vi "GDFreadData.vi"(0 "GDFv1.x.lvclass in":refnum<class "GDFv1.x.lvclass">, 9 "Channel Number":i64, 11 "error in":errorcluster) -> (4 "GDFv1.x.lvclass out":refnum<class "GDFv1.x.lvclass">, 6 "waveform out":waveform(dbl), 15 "error out":errorcluster)   [LabVIEW 2016, in "GDF File Reader.lvlib" / "GDFv1.x.lvclass"]
uses:
  GDFv1.x.lvclass
  GDFv1.x.lvclass/GDFv1.x.ctl
panel:
  # "This VI is a part of BCI Design library, http://www.ru-bci.org \nCopyright © 2020, Sotnikov Peter, All rights reserved. License: CC BY-NC 4.0"
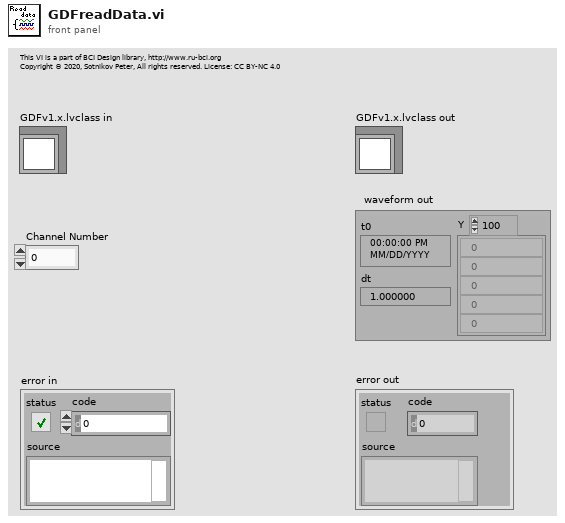
[diagram p1: front panel]
types:
  T1 = typedef "GDF File Reader.lvlib/GdfHeader1.ctl" = cluster{"Version identificator":string, "Patient identificator":string, "Recording identificator":string, "StartDateTime":timestamp, "Header record length":i64, "Equipment Provider":u64, "Laboratory":u64, "Technician":u64, "Number of data records":i64, "Duration of a data record":cluster{"Numerator":u32, "Denominator":u32}, "Number of signals":u32}
  T2 = typedef "GDF File Reader.lvlib/GdfHeader2.ctl" = cluster{"Channel labels":string[], "Transduser types":string[], "Physical dimensions":string[], "Physical lows":dbl[], "Physical highs":dbl[], "Digital lows":dbl[], "Digital highs":dbl[], "Channels Pre-filtering":string[], "Number of samples":u32[], "Channel types":u32[], "Addons":string[]}
  T3 = enum16{"big-endian, network order", "native, host order", "little-endian"}
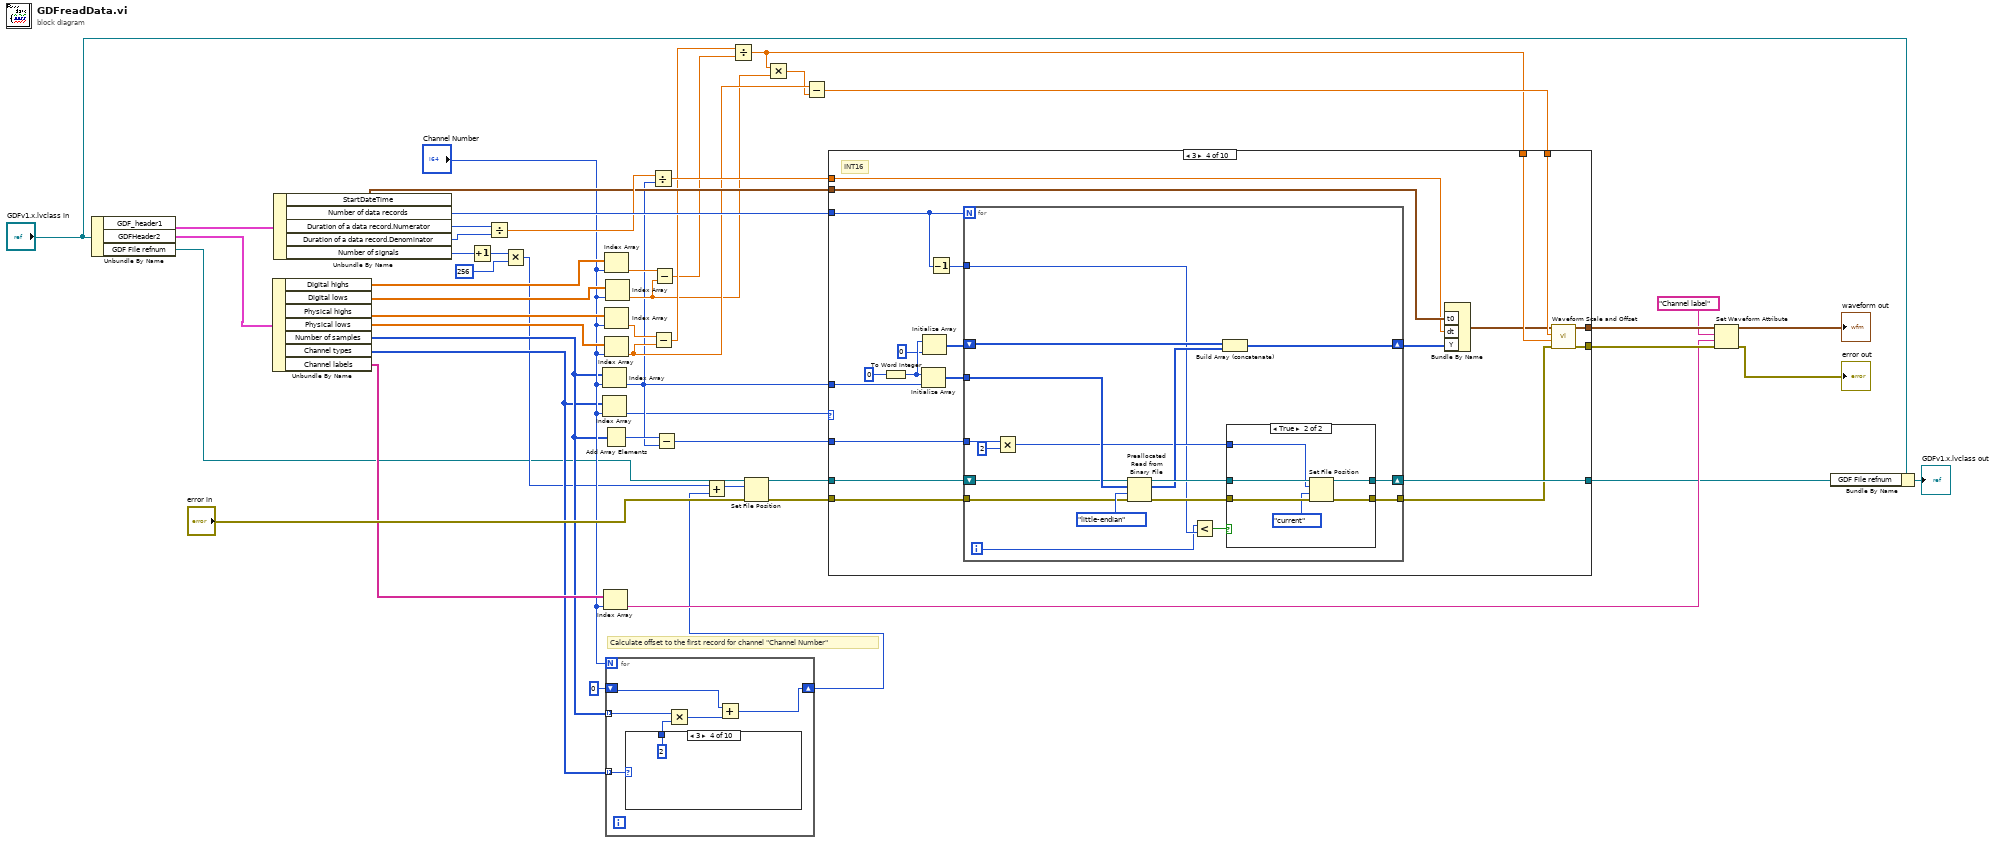
[diagram p0: block diagram]
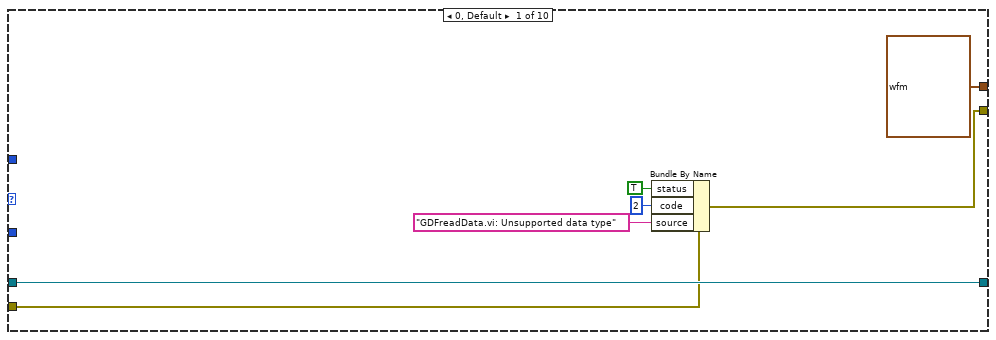
[diagram p2: hidden frame]
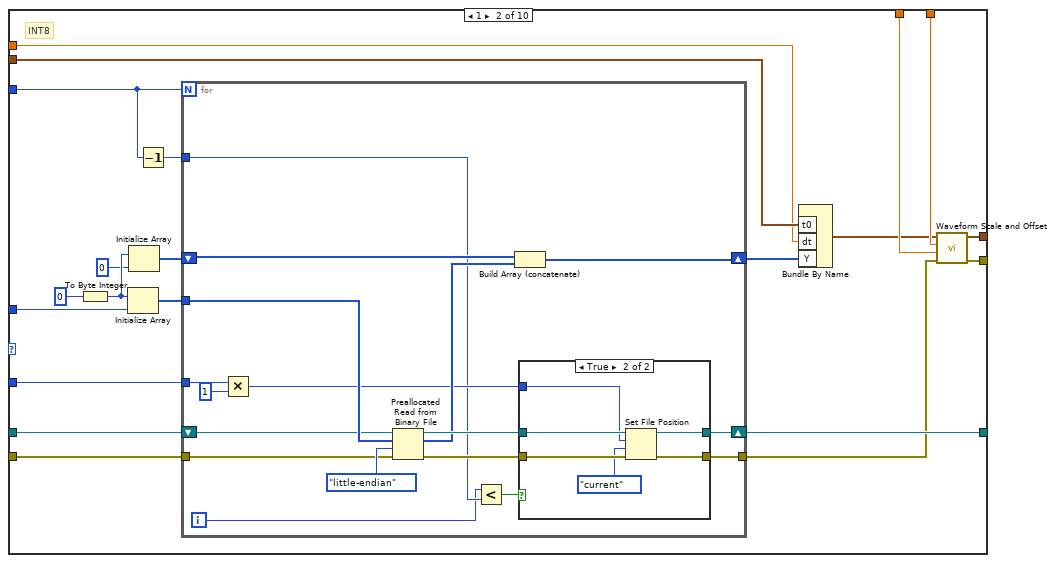
[diagram p3: hidden frame]
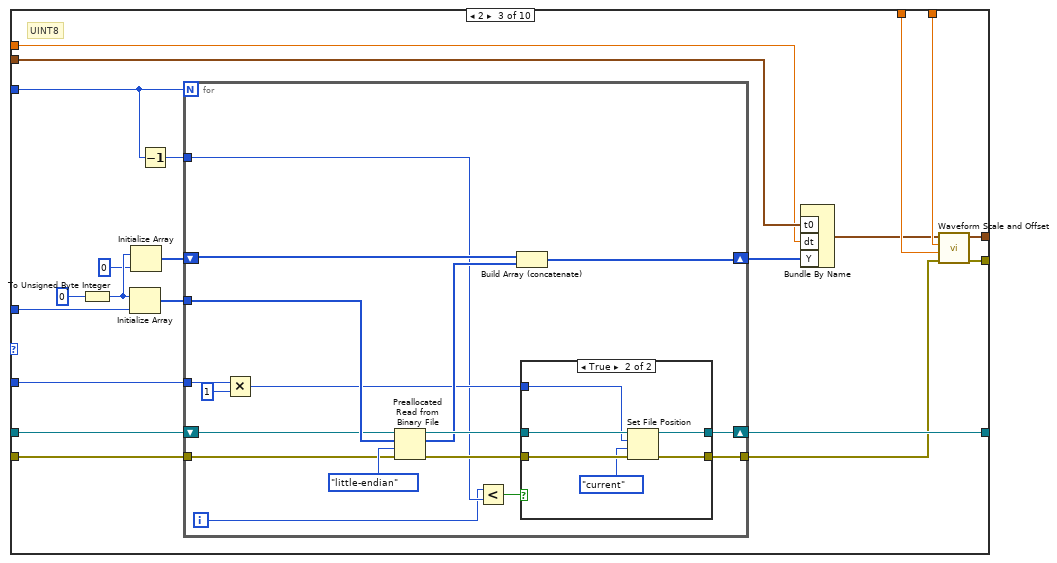
[diagram p5: hidden frame]
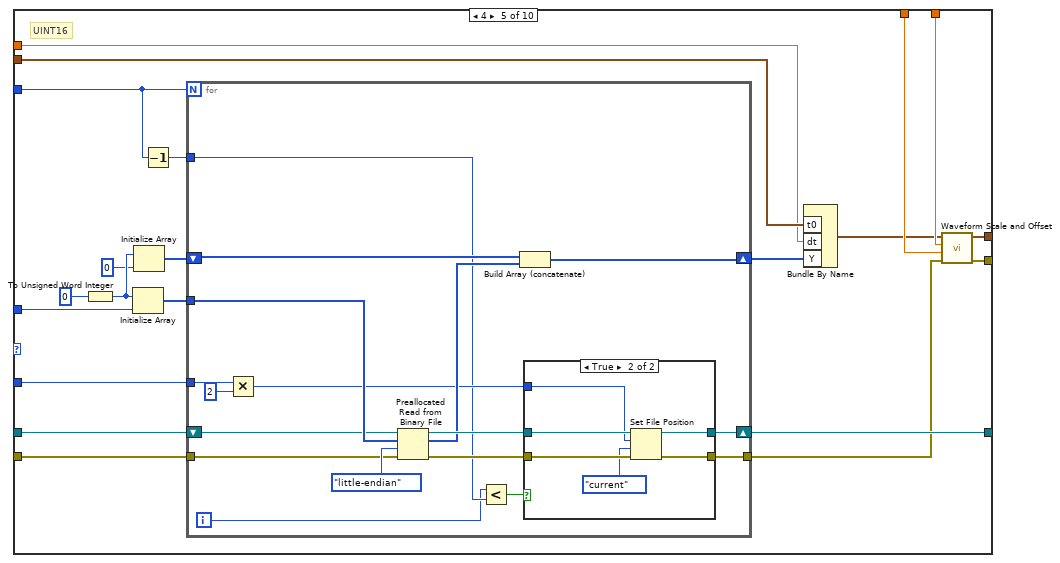
[diagram p8: hidden frame]
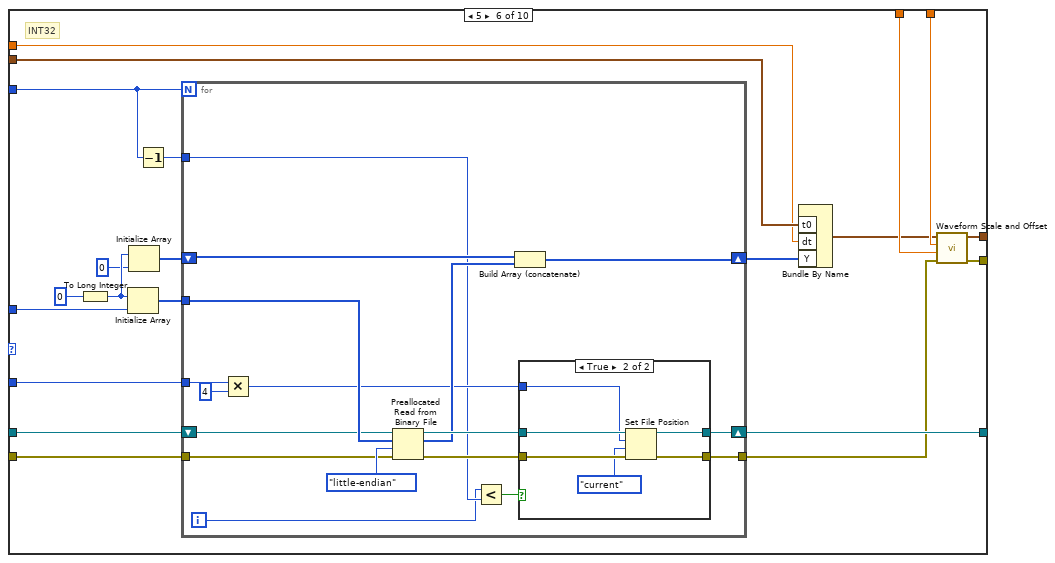
[diagram p10: hidden frame]
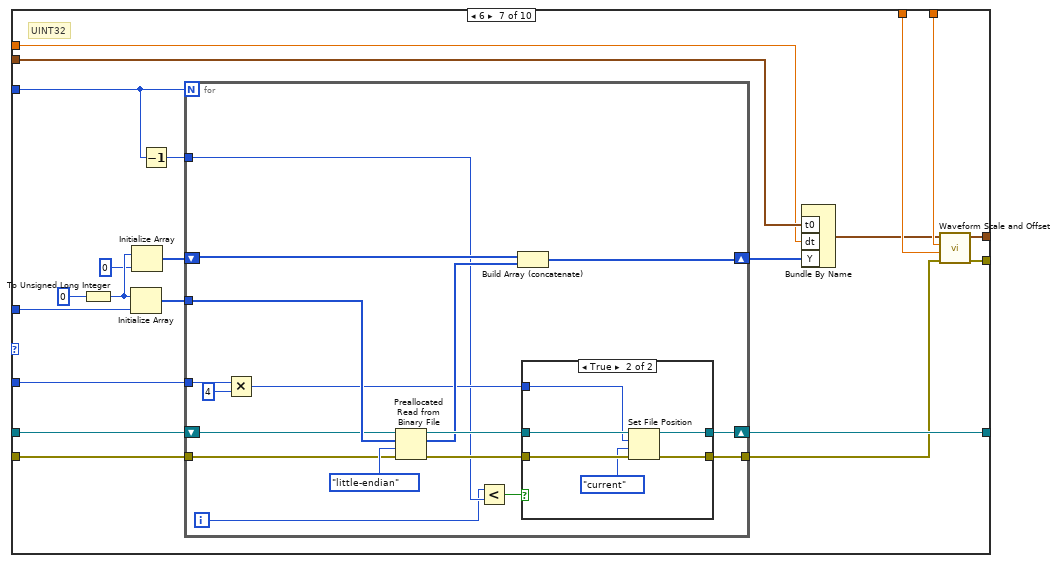
[diagram p12: hidden frame]
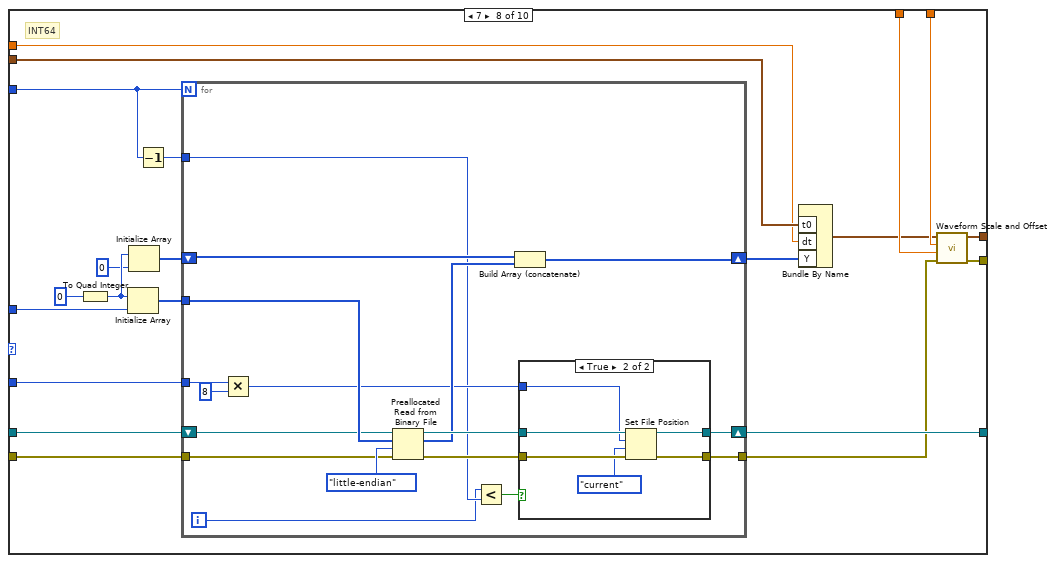
[diagram p14: hidden frame]
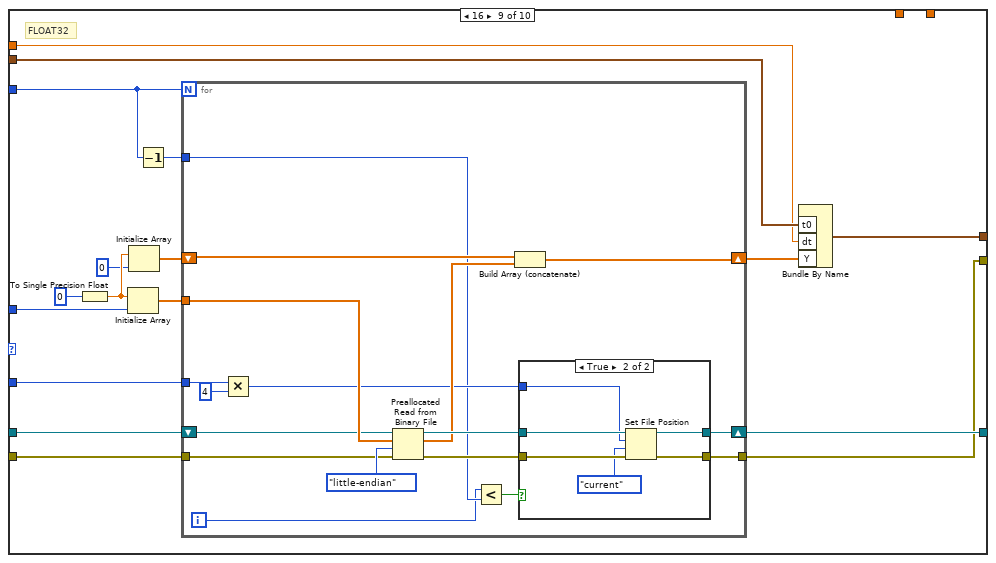
[diagram p16: hidden frame]
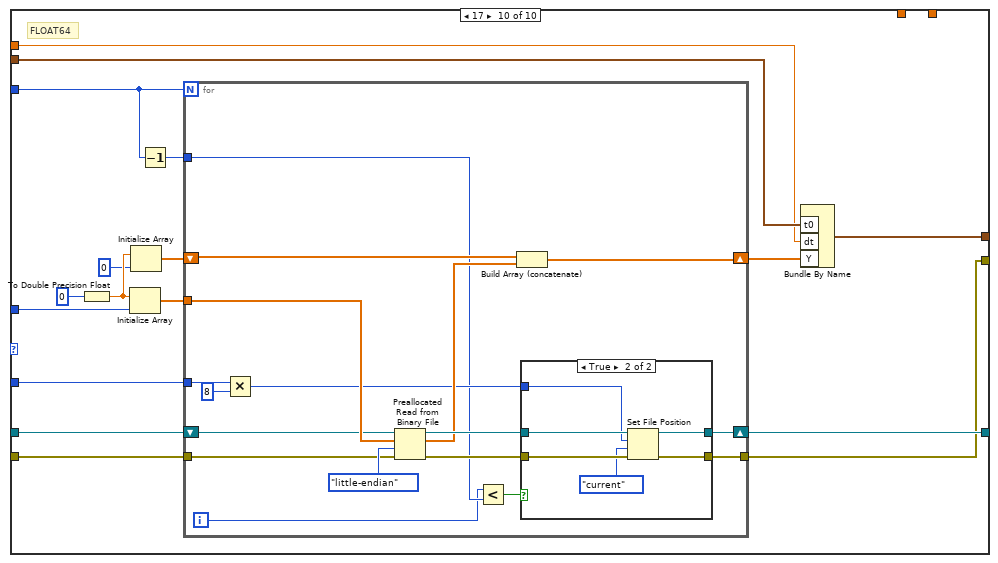
[diagram p18: hidden frame]
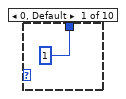
[diagram p20: hidden frame]
diagram:
  # "Calculate offset to the first record for channel \"Channel Number\""
  n1 = Unbundle By Name("GDFv1.x.lvclass in") -> ("GDF_header1"=w6:T1, "GDFHeader2"=w5:T2, "GDF File refnum"=w4:refnum<file>)
  n2 = Unbundle By Name(w5) -> ("Digital highs"=w43:dbl[], "Digital lows"=w33:dbl[], "Physical highs"=w44:dbl[], "Physical lows"=w45:dbl[], "Number of samples"=w14:u32[], "Channel types"=w13:u32[], "Channel labels"=w18:string[])
  n3 = Unbundle By Name(w6) -> ("StartDateTime"=w36:timestamp, "Number of data records"=w46:i64, "Duration of a data record.Numerator"=w39:u32, "Duration of a data record.Denominator"=w38:u32, "Number of signals"=w47:u32)
  n4 = Increment(x=w47) -> (x+1=w49:u32)
  n5 = Divide(x=w39, y=w38) -> (x/y=w37:dbl)
  n6 = Multiply(x=w49, y=u32 256) -> (x*y=w11:u32)
  n7 = Index Array(array=w14, index="Channel Number") -> (element=w23:u32)
  n8 = Index Array(array=w13, index="Channel Number") -> (element=w7:u32)
  n9 = Index Array(array=w18, index="Channel Number") -> (element=w17:string)
  n10 = Index Array(array=w45, index="Channel Number") -> (element=w29:dbl)
  n11 = Add Array Elements(numeric array=w14) -> (sum=w24:u32)
  n12 = Index Array(array=w43, index="Channel Number") -> (element=w32:dbl)
  n13 = Index Array(array=w44, index="Channel Number") -> (element=w34:dbl)
  n14 = Index Array(array=w33, index="Channel Number") -> (element=w27:dbl)
  n15 = for {
    N: "Channel Number" -> [_]
    tunnel: w14 -> [w54] mode=indexing
    tunnel: w13 -> [w55] mode=indexing
    shift-right: [w50] -> w10
    shift-left: u32 0 -> [w51]
    n16 = case shown="3" w55 {
      tunnel: [1 1 1 2 2 4 4 8 4 8] -> w53
      frame 0, Default {
      }
      frame 1 {
      }
      frame 2 {
      }
      frame 3 {
      }
      frame 4 {
      }
      frame 5 {
      }
      frame 6 {
      }
      frame 7 {
      }
      frame 16 {
      }
      frame 17 {
      }
    }
    n17 = Multiply(x=w54, y=w53) -> (x*y=w52:u32)
    n18 = Add(x=w51, y=w52) -> (x+y=w50:u32)
  }
  n19 = Divide(x=w37, y=w23) -> (x/y=w35:dbl)
  n20 = Subtract(x=w34, y=w29) -> (x-y=w31:dbl)
  n21 = Subtract(x=w32, y=w27) -> (x-y=w30:dbl)
  n22 = Subtract(x=w24, y=w23) -> (x-y=w22:u32)
  n23 = Add(x=w11, y=w10) -> (x+y=w9:u32)
  n24 = Divide(x=w31, y=w30) -> (x/y=w25:dbl)
  n25 = Set File Position(offset (in bytes) (0)=w9, refnum=w4, error in="error in") -> (refnum out=w40:refnum<file>, error out=w41:errorcluster)  [unwired: 1 in]
  n26 = Multiply(x=w25, y=w27) -> (x*y=w28:dbl)
  n27 = Subtract(x=w29, y=w28) -> (x-y=w26:dbl)
  n28 = case shown="3" w7 {
    tunnel: w46 -> [_ w93 w139 w185 w231 w277 w323 w369 w411 w453]
    tunnel: w41 -> [w70 w92 w138 w184 w230 w276 w322 w368 w410 w452]
    tunnel: w40 -> [w71 w91 w137 w183 w229 w275 w321 w367 w409 w451]
    tunnel: [w71 w90 w136 w182 w228 w274 w320 w366 w408 w450] -> w2
    tunnel: w36 -> [_ w89 w135 w181 w227 w273 w319 w365 w407 w449]
    tunnel: w35 -> [_ w88 w134 w180 w226 w272 w318 w364 w406 w448]
    tunnel: w26 -> [_ w87 w133 w179 w225 w271 w317 w363 _ _]
    tunnel: w25 -> [_ w86 w132 w178 w224 w270 w316 w362 _ _]
    tunnel: w23 -> [_ w85 w131 w177 w223 w269 w315 w361 w405 w447]
    tunnel: w22 -> [_ w84 w130 w176 w222 w268 w314 w360 w404 w446]
    tunnel: [waveform(dbl) {"t0"=timestamp(0 s since 1904-01-01), "dt"=1.0, "Y"=[]} ("waveform out") w83 w129 w175 w221 w267 w313 w359 w396 w438] -> w21
    tunnel: [w69 w82 w128 w174 w220 w266 w312 w358 w395 w437] -> w20
    frame 0, Default {
      n29 = Bundle By Name(cluster=w70, "status"=TRUE, "code"=2, "source"="GDFreadData.vi: Unsupported data type") -> (w69:errorcluster)
    }
    frame 1 {
      # "INT8"
      n30 = To Byte Integer(number=i16 0) -> (8bit integer=w77:i8)
      n31 = Initialize Array(w77, w85) -> (w78:i8[])
      n32 = Initialize Array(w77, 0 ("dimension size")) -> (w76:i8[])
      n33 = Decrement(x=w93) -> (x-1=w73:i64)
      n34 = for {
        N: w93 -> [_]
        tunnel: w78 -> [w110]
        tunnel: w92 -> [w108]
        tunnel: [w104] -> w80
        shift-right: [w103] -> w90
        shift-left: w91 -> [w107]
        shift-right: [w101] -> w74
        shift-left: w76 -> [w100]
        tunnel: w84 -> [w99]
        tunnel: w73 -> [w95]
        i -> [w94]
        n35 = Multiply(x=w99, y=u32 1) -> (x*y=w97:u32)
        n36 = Preallocated Read from Binary File(4:w108, 5:T3."little-endian" ("byte order (0:big-endian, network order)"), 6:w110, 7:w107) -> (0:w106:errorcluster, 2:w102:i8[], 3:w105:refnum<file>)  [unwired: 1 out]
        n37 = Less?(x=w94, y=w95) -> (x < y?=w96:bool)
        n38 = Build Array (concatenate)(w100, w102) -> (w101:i8[])
        n39 = case shown="True" w96 {
          tunnel: w106 -> [w111 w118]
          tunnel: w105 -> [w112 w117]
          tunnel: [w111 w115] -> w104
          tunnel: [w112 w114] -> w103
          tunnel: w97 -> [_ w113]
          frame False {
          }
          frame True {
            n40 = Set File Position(offset (in bytes) (0)=w113, refnum=w117, from (0:start)=enum16{"start", "end", "current"}."current", error in=w118) -> (refnum out=w114:refnum<file>, error out=w115:errorcluster)
          }
        }
      }
      n41 = Bundle By Name("t0"=w89, "dt"=w88, "Y"=w74) -> (w81:waveform(i8))  [unwired: 1 in]
      n42 = call <vilib>:"Waveform Scale and Offset.vi"("error in (no error)"=w80, "scale"=w86, "offset"=w87, "waveform in"=w81) -> ("error out"=w82:errorcluster, "waveform out"=w83:waveform(dbl))  [unwired: 6 in]
    }
    frame 2 {
      # "UINT8"
      n43 = To Unsigned Byte Integer(number=i16 0) -> (unsigned 8bit integer=w123:u8)
      n44 = Initialize Array(w123, w131) -> (w124:u8[])
      n45 = Initialize Array(w123, 0 ("dimension size")) -> (w122:u8[])
      n46 = Decrement(x=w139) -> (x-1=w119:i64)
      n47 = for {
        N: w139 -> [_]
        tunnel: w124 -> [w156]
        tunnel: w138 -> [w154]
        tunnel: [w150] -> w126
        shift-right: [w149] -> w136
        shift-left: w137 -> [w153]
        shift-right: [w147] -> w120
        shift-left: w122 -> [w146]
        tunnel: w130 -> [w145]
        tunnel: w119 -> [w141]
        i -> [w140]
        n48 = Multiply(x=w145, y=u32 1) -> (x*y=w143:u32)
        n49 = Preallocated Read from Binary File(4:w154, 5:T3."little-endian" ("byte order (0:big-endian, network order)"), 6:w156, 7:w153) -> (0:w152:errorcluster, 2:w148:u8[], 3:w151:refnum<file>)  [unwired: 1 out]
        n50 = Less?(x=w140, y=w141) -> (x < y?=w142:bool)
        n51 = Build Array (concatenate)(w146, w148) -> (w147:u8[])
        n52 = case shown="True" w142 {
          tunnel: w152 -> [w157 w164]
          tunnel: w151 -> [w158 w163]
          tunnel: [w157 w161] -> w150
          tunnel: [w158 w160] -> w149
          tunnel: w143 -> [_ w159]
          frame False {
          }
          frame True {
            n53 = Set File Position(offset (in bytes) (0)=w159, refnum=w163, from (0:start)=enum16{"start", "end", "current"}."current", error in=w164) -> (refnum out=w160:refnum<file>, error out=w161:errorcluster)
          }
        }
      }
      n54 = Bundle By Name("t0"=w135, "dt"=w134, "Y"=w120) -> (w127:waveform(u8))  [unwired: 1 in]
      n55 = call <vilib>:"Waveform Scale and Offset.vi"("error in (no error)"=w126, "scale"=w132, "offset"=w133, "waveform in"=w127) -> ("error out"=w128:errorcluster, "waveform out"=w129:waveform(dbl))  [unwired: 6 in]
    }
    frame 3 {
      # "INT16"
      n56 = To Word Integer(number=i16 0) -> (16bit integer=w169:i16)
      n57 = Initialize Array(w169, w177) -> (w170:i16[])
      n58 = Initialize Array(w169, 0 ("dimension size")) -> (w168:i16[])
      n59 = Decrement(x=w185) -> (x-1=w165:i64)
      n60 = for {
        N: w185 -> [_]
        tunnel: w170 -> [w202]
        tunnel: w184 -> [w200]
        tunnel: [w196] -> w172
        shift-right: [w195] -> w182
        shift-left: w183 -> [w199]
        shift-right: [w193] -> w166
        shift-left: w168 -> [w192]
        tunnel: w176 -> [w191]
        tunnel: w165 -> [w187]
        i -> [w186]
        n61 = Multiply(x=w191, y=u32 2) -> (x*y=w189:u32)
        n62 = Preallocated Read from Binary File(4:w200, 5:T3."little-endian" ("byte order (0:big-endian, network order)"), 6:w202, 7:w199) -> (0:w198:errorcluster, 2:w194:i16[], 3:w197:refnum<file>)  [unwired: 1 out]
        n63 = Less?(x=w186, y=w187) -> (x < y?=w188:bool)
        n64 = Build Array (concatenate)(w192, w194) -> (w193:i16[])
        n65 = case shown="True" w188 {
          tunnel: w198 -> [w203 w210]
          tunnel: w197 -> [w204 w209]
          tunnel: [w203 w207] -> w196
          tunnel: [w204 w206] -> w195
          tunnel: w189 -> [_ w205]
          frame False {
          }
          frame True {
            n66 = Set File Position(offset (in bytes) (0)=w205, refnum=w209, from (0:start)=enum16{"start", "end", "current"}."current", error in=w210) -> (refnum out=w206:refnum<file>, error out=w207:errorcluster)
          }
        }
      }
      n67 = Bundle By Name("t0"=w181, "dt"=w180, "Y"=w166) -> (w173:waveform(i16))  [unwired: 1 in]
      n68 = call <vilib>:"Waveform Scale and Offset.vi"("error in (no error)"=w172, "scale"=w178, "offset"=w179, "waveform in"=w173) -> ("error out"=w174:errorcluster, "waveform out"=w175:waveform(dbl))  [unwired: 6 in]
    }
    frame 4 {
      # "UINT16"
      n69 = To Unsigned Word Integer(number=i16 0) -> (unsigned 16bit integer=w215:u16)
      n70 = Initialize Array(w215, w223) -> (w216:u16[])
      n71 = Initialize Array(w215, 0 ("dimension size")) -> (w214:u16[])
      n72 = Decrement(x=w231) -> (x-1=w211:i64)
      n73 = for {
        N: w231 -> [_]
        tunnel: w216 -> [w248]
        tunnel: w230 -> [w246]
        tunnel: [w242] -> w218
        shift-right: [w241] -> w228
        shift-left: w229 -> [w245]
        shift-right: [w239] -> w212
        shift-left: w214 -> [w238]
        tunnel: w222 -> [w237]
        tunnel: w211 -> [w233]
        i -> [w232]
        n74 = Multiply(x=w237, y=u32 2) -> (x*y=w235:u32)
        n75 = Preallocated Read from Binary File(4:w246, 5:T3."little-endian" ("byte order (0:big-endian, network order)"), 6:w248, 7:w245) -> (0:w244:errorcluster, 2:w240:u16[], 3:w243:refnum<file>)  [unwired: 1 out]
        n76 = Less?(x=w232, y=w233) -> (x < y?=w234:bool)
        n77 = Build Array (concatenate)(w238, w240) -> (w239:u16[])
        n78 = case shown="True" w234 {
          tunnel: w244 -> [w249 w256]
          tunnel: w243 -> [w250 w255]
          tunnel: [w249 w253] -> w242
          tunnel: [w250 w252] -> w241
          tunnel: w235 -> [_ w251]
          frame False {
          }
          frame True {
            n79 = Set File Position(offset (in bytes) (0)=w251, refnum=w255, from (0:start)=enum16{"start", "end", "current"}."current", error in=w256) -> (refnum out=w252:refnum<file>, error out=w253:errorcluster)
          }
        }
      }
      n80 = Bundle By Name("t0"=w227, "dt"=w226, "Y"=w212) -> (w219:waveform(u16))  [unwired: 1 in]
      n81 = call <vilib>:"Waveform Scale and Offset.vi"("error in (no error)"=w218, "scale"=w224, "offset"=w225, "waveform in"=w219) -> ("error out"=w220:errorcluster, "waveform out"=w221:waveform(dbl))  [unwired: 6 in]
    }
    frame 5 {
      # "INT32"
      n82 = To Long Integer(number=i16 0) -> (32bit integer=w261:i32)
      n83 = Initialize Array(w261, w269) -> (w262:i32[])
      n84 = Initialize Array(w261, 0 ("dimension size")) -> (w260:i32[])
      n85 = Decrement(x=w277) -> (x-1=w257:i64)
      n86 = for {
        N: w277 -> [_]
        tunnel: w262 -> [w294]
        tunnel: w276 -> [w292]
        tunnel: [w288] -> w264
        shift-right: [w287] -> w274
        shift-left: w275 -> [w291]
        shift-right: [w285] -> w258
        shift-left: w260 -> [w284]
        tunnel: w268 -> [w283]
        tunnel: w257 -> [w279]
        i -> [w278]
        n87 = Multiply(x=w283, y=u32 4) -> (x*y=w281:u32)
        n88 = Preallocated Read from Binary File(4:w292, 5:T3."little-endian" ("byte order (0:big-endian, network order)"), 6:w294, 7:w291) -> (0:w290:errorcluster, 2:w286:i32[], 3:w289:refnum<file>)  [unwired: 1 out]
        n89 = Less?(x=w278, y=w279) -> (x < y?=w280:bool)
        n90 = Build Array (concatenate)(w284, w286) -> (w285:i32[])
        n91 = case shown="True" w280 {
          tunnel: w290 -> [w295 w302]
          tunnel: w289 -> [w296 w301]
          tunnel: [w295 w299] -> w288
          tunnel: [w296 w298] -> w287
          tunnel: w281 -> [_ w297]
          frame False {
          }
          frame True {
            n92 = Set File Position(offset (in bytes) (0)=w297, refnum=w301, from (0:start)=enum16{"start", "end", "current"}."current", error in=w302) -> (refnum out=w298:refnum<file>, error out=w299:errorcluster)
          }
        }
      }
      n93 = Bundle By Name("t0"=w273, "dt"=w272, "Y"=w258) -> (w265:waveform(i32))  [unwired: 1 in]
      n94 = call <vilib>:"Waveform Scale and Offset.vi"("error in (no error)"=w264, "scale"=w270, "offset"=w271, "waveform in"=w265) -> ("error out"=w266:errorcluster, "waveform out"=w267:waveform(dbl))  [unwired: 6 in]
    }
    frame 6 {
      # "UINT32"
      n95 = To Unsigned Long Integer(number=i16 0) -> (unsigned 32bit integer=w307:u32)
      n96 = Initialize Array(w307, w315) -> (w308:u32[])
      n97 = Initialize Array(w307, 0 ("dimension size")) -> (w306:u32[])
      n98 = Decrement(x=w323) -> (x-1=w303:i64)
      n99 = for {
        N: w323 -> [_]
        tunnel: w308 -> [w340]
        tunnel: w322 -> [w338]
        tunnel: [w334] -> w310
        shift-right: [w333] -> w320
        shift-left: w321 -> [w337]
        shift-right: [w331] -> w304
        shift-left: w306 -> [w330]
        tunnel: w314 -> [w329]
        tunnel: w303 -> [w325]
        i -> [w324]
        n100 = Multiply(x=w329, y=u32 4) -> (x*y=w327:u32)
        n101 = Preallocated Read from Binary File(4:w338, 5:T3."little-endian" ("byte order (0:big-endian, network order)"), 6:w340, 7:w337) -> (0:w336:errorcluster, 2:w332:u32[], 3:w335:refnum<file>)  [unwired: 1 out]
        n102 = Less?(x=w324, y=w325) -> (x < y?=w326:bool)
        n103 = Build Array (concatenate)(w330, w332) -> (w331:u32[])
        n104 = case shown="True" w326 {
          tunnel: w336 -> [w341 w348]
          tunnel: w335 -> [w342 w347]
          tunnel: [w341 w345] -> w334
          tunnel: [w342 w344] -> w333
          tunnel: w327 -> [_ w343]
          frame False {
          }
          frame True {
            n105 = Set File Position(offset (in bytes) (0)=w343, refnum=w347, from (0:start)=enum16{"start", "end", "current"}."current", error in=w348) -> (refnum out=w344:refnum<file>, error out=w345:errorcluster)
          }
        }
      }
      n106 = Bundle By Name("t0"=w319, "dt"=w318, "Y"=w304) -> (w311:waveform(u32))  [unwired: 1 in]
      n107 = call <vilib>:"Waveform Scale and Offset.vi"("error in (no error)"=w310, "scale"=w316, "offset"=w317, "waveform in"=w311) -> ("error out"=w312:errorcluster, "waveform out"=w313:waveform(dbl))  [unwired: 6 in]
    }
    frame 7 {
      # "INT64"
      n108 = To Quad Integer(1:i16 0 ("number")) -> (0:w353:i64)
      n109 = Initialize Array(w353, w361) -> (w354:i64[])
      n110 = Initialize Array(w353, 0 ("dimension size")) -> (w352:i64[])
      n111 = Decrement(x=w369) -> (x-1=w349:i64)
      n112 = for {
        N: w369 -> [_]
        tunnel: w354 -> [w386]
        tunnel: w368 -> [w384]
        tunnel: [w380] -> w356
        shift-right: [w379] -> w366
        shift-left: w367 -> [w383]
        shift-right: [w377] -> w350
        shift-left: w352 -> [w376]
        tunnel: w360 -> [w375]
        tunnel: w349 -> [w371]
        i -> [w370]
        n113 = Multiply(x=w375, y=u32 8) -> (x*y=w373:u32)
        n114 = Preallocated Read from Binary File(4:w384, 5:T3."little-endian" ("byte order (0:big-endian, network order)"), 6:w386, 7:w383) -> (0:w382:errorcluster, 2:w378:i64[], 3:w381:refnum<file>)  [unwired: 1 out]
        n115 = Less?(x=w370, y=w371) -> (x < y?=w372:bool)
        n116 = Build Array (concatenate)(w376, w378) -> (w377:i64[])
        n117 = case shown="True" w372 {
          tunnel: w382 -> [w387 w394]
          tunnel: w381 -> [w388 w393]
          tunnel: [w387 w391] -> w380
          tunnel: [w388 w390] -> w379
          tunnel: w373 -> [_ w389]
          frame False {
          }
          frame True {
            n118 = Set File Position(offset (in bytes) (0)=w389, refnum=w393, from (0:start)=enum16{"start", "end", "current"}."current", error in=w394) -> (refnum out=w390:refnum<file>, error out=w391:errorcluster)
          }
        }
      }
      n119 = Bundle By Name("t0"=w365, "dt"=w364, "Y"=w350) -> (w357:waveform(i64))  [unwired: 1 in]
      n120 = call <vilib>:"Waveform Scale and Offset.vi"("error in (no error)"=w356, "scale"=w362, "offset"=w363, "waveform in"=w357) -> ("error out"=w358:errorcluster, "waveform out"=w359:waveform(dbl))  [unwired: 6 in]
    }
    frame 16 {
      # "FLOAT32"
      n121 = To Single Precision Float(number=i16 0) -> (single precision float=w401:sgl)
      n122 = Initialize Array(w401, w405) -> (w402:sgl[])
      n123 = Initialize Array(w401, 0 ("dimension size")) -> (w400:sgl[])
      n124 = Decrement(x=w411) -> (x-1=w397:i64)
      n125 = for {
        N: w411 -> [_]
        tunnel: w402 -> [w428]
        tunnel: w410 -> [w426]
        tunnel: [w422] -> w395
        shift-right: [w421] -> w408
        shift-left: w409 -> [w425]
        shift-right: [w419] -> w398
        shift-left: w400 -> [w418]
        tunnel: w404 -> [w417]
        tunnel: w397 -> [w413]
        i -> [w412]
        n126 = Multiply(x=w417, y=u32 4) -> (x*y=w415:u32)
        n127 = Preallocated Read from Binary File(4:w426, 5:T3."little-endian" ("byte order (0:big-endian, network order)"), 6:w428, 7:w425) -> (0:w424:errorcluster, 2:w420:sgl[], 3:w423:refnum<file>)  [unwired: 1 out]
        n128 = Less?(x=w412, y=w413) -> (x < y?=w414:bool)
        n129 = Build Array (concatenate)(w418, w420) -> (w419:sgl[])
        n130 = case shown="True" w414 {
          tunnel: w424 -> [w429 w436]
          tunnel: w423 -> [w430 w435]
          tunnel: [w429 w433] -> w422
          tunnel: [w430 w432] -> w421
          tunnel: w415 -> [_ w431]
          frame False {
          }
          frame True {
            n131 = Set File Position(offset (in bytes) (0)=w431, refnum=w435, from (0:start)=enum16{"start", "end", "current"}."current", error in=w436) -> (refnum out=w432:refnum<file>, error out=w433:errorcluster)
          }
        }
      }
      n132 = Bundle By Name("t0"=w407, "dt"=w406, "Y"=w398) -> (w396:waveform(sgl))  [unwired: 1 in]
    }
    frame 17 {
      # "FLOAT64"
      n133 = To Double Precision Float(number=i16 0) -> (double precision float=w443:dbl)
      n134 = Initialize Array(w443, w447) -> (w444:dbl[])
      n135 = Initialize Array(w443, 0 ("dimension size")) -> (w442:dbl[])
      n136 = Decrement(x=w453) -> (x-1=w439:i64)
      n137 = for {
        N: w453 -> [_]
        tunnel: w444 -> [w470]
        tunnel: w452 -> [w468]
        tunnel: [w464] -> w437
        shift-right: [w463] -> w450
        shift-left: w451 -> [w467]
        shift-right: [w461] -> w440
        shift-left: w442 -> [w460]
        tunnel: w446 -> [w459]
        tunnel: w439 -> [w455]
        i -> [w454]
        n138 = Multiply(x=w459, y=u32 8) -> (x*y=w457:u32)
        n139 = Preallocated Read from Binary File(4:w468, 5:T3."little-endian" ("byte order (0:big-endian, network order)"), 6:w470, 7:w467) -> (0:w466:errorcluster, 2:w462:dbl[], 3:w465:refnum<file>)  [unwired: 1 out]
        n140 = Less?(x=w454, y=w455) -> (x < y?=w456:bool)
        n141 = Build Array (concatenate)(w460, w462) -> (w461:dbl[])
        n142 = case shown="True" w456 {
          tunnel: w466 -> [w471 w478]
          tunnel: w465 -> [w472 w477]
          tunnel: [w471 w475] -> w464
          tunnel: [w472 w474] -> w463
          tunnel: w457 -> [_ w473]
          frame False {
          }
          frame True {
            n143 = Set File Position(offset (in bytes) (0)=w473, refnum=w477, from (0:start)=enum16{"start", "end", "current"}."current", error in=w478) -> (refnum out=w474:refnum<file>, error out=w475:errorcluster)
          }
        }
      }
      n144 = Bundle By Name("t0"=w449, "dt"=w448, "Y"=w440) -> (w438:waveform(dbl))  [unwired: 1 in]
    }
  }
  n145 = Set Waveform Attribute(4:w20, 5:w17, 6:"Channel label" ("name"), 7:w21) -> (0:→"error out":errorcluster, 3:→"waveform out":waveform(dbl))  [unwired: 1 out]
  n146 = Bundle By Name(cluster="GDFv1.x.lvclass in", "GDF File refnum"=w2) -> (→"GDFv1.x.lvclass out":refnum<class "GDFv1.x.lvclass">)
